vi "Heel Strike VI.vi"(3 "all rows":dbl[](array[numeric])) -> (0 "Heel Strike":i32[](array[numeric]), 1 "Heel FSR":cluster{"Indices":i32[], "all rows":dbl[]}[](array[cluster]))   [LabVIEW 2021]
uses:
  <vilib>/Analysis/NI_AALPro.lvlib
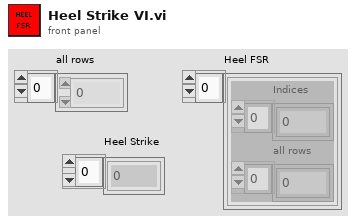
[diagram p1: front panel]
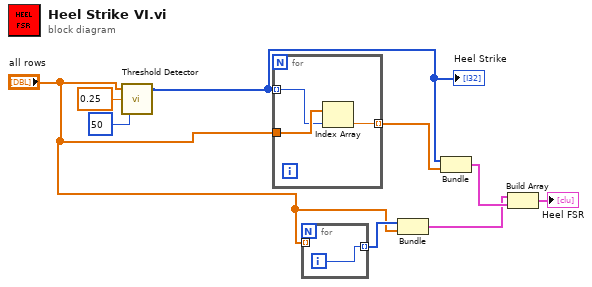
[diagram p0: block diagram]
diagram:
  n1 = call <vilib>:"Threshold Detector.vi"("width"=50, "threshold"=0.25, "X"="all rows") -> ("Indices"=w4:i32[])  [unwired: 2 out]
  "Heel Strike" <- w4
  n2 = for {
    tunnel: w4 -> [w11] mode=indexing
    tunnel: "all rows" -> [w12]
    tunnel: [w10] -> w3 mode=indexing
    n3 = Index Array(array=w12, index=w11) -> (element=w10:dbl)
  }
  n4 = for {
    tunnel: "all rows" -> [_] mode=indexing
    tunnel: [w13] -> w6 mode=indexing
    i -> [w13]
  }
  n5 = Bundle(w6, "all rows"="all rows") -> (w7:cluster{i32[], "all rows":dbl[]})  [unwired: 1 in]
  n6 = Bundle("Indices"=w4, w3) -> (w8:cluster{"Indices":i32[], dbl[]})  [unwired: 1 in]
  n7 = Build Array(w7, w8) -> (→"Heel FSR":cluster{"Indices":i32[], "all rows":dbl[]}[])
